vi "SatelliteTracking.vi"() -> ()   [LabVIEW 2014]
uses:
  <vilib>/Analysis/NI_AALBase.lvlib
  <vilib>/measure/NI_MAPro.lvlib
  <vilib>/measure/maspectr.llb/FFT Power Spectrum and PSD for 1 Chan.vi
  <vilib>/Analysis/4window.llb/windowTd.ctl
  <vilib>/Analysis/NI_AALPro.lvlib
panel:
  in  "dB On (F)":bool
  in  "window parameter":dbl=nan
  in  "window":T1=1 items=["Rectangle"=0, "Hanning"=1, "Hamming"=2, "Blackman-Harris"=3, "Exact Blackman"=4, "Blackman"=5, "Flat Top"=6, "4 Term B-Harris "=7, "7 Term B-Harris"=8, "Low Sidelobe"=9, "Blackman Nuttall"=11, "Triangle"=30, "Bartlett-Hanning"=31, "Bohman"=32, "Parzen"=33, "Welch"=34, "Kaiser"=60, "Dolph-Chebyshev"=61, "Gaussian"=62]
  in  "averaging parameters":T2={"averaging mode"=enum."No averaging", "weighting mode"=enum."Exponential", "number of averages"=10} {"number of averages" min=1}
  out "Power Spectrum":cluster{"f0":dbl, "df":dbl, "magnitude":dbl[]}(graph)
  in  "frequency":dbl=0.0078125 format="%0.4e"
  in  "amplitude":dbl=1.0 format="%0.2f"
  in  "samples":i32=128
  in  "Longitude":dbl=-1.307 format="%#.6g"
  in  "Latitude":dbl=51.4062 format="%#.6g"
  out "URL":string="http://maps.google.com/staticmap?center=51.406200,-1.307000&zoom=18&size=570x350&maptype=hybrid&markers=51.406200,-1.307000,midpurplea&key=&path=rgb:0xFF1000,weight:5|51.406200,-1.307000|51.406200,-1.307000"
  in  "?":refnum<k7>(container)
  # "Start Position"
  # "Balloon Position"
  # "This is an 86 character alphanumeric key supplied by Google"
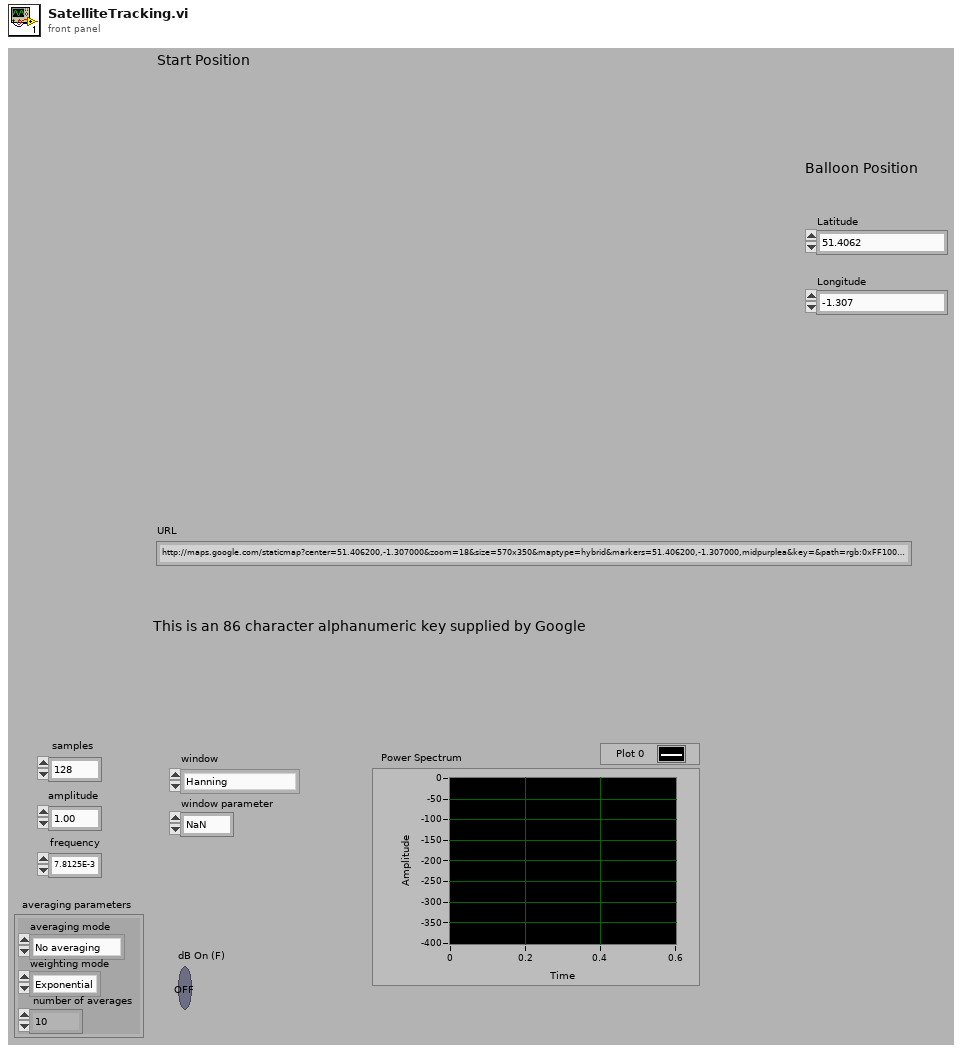
[diagram p1: front panel]
types:
  T1 = typedef "NI_AALPro.lvlib/windowTd.ctl" = u32
  T2 = cluster{"averaging mode":enum16{"No averaging", "Vector averaging", "RMS averaging", "Peak hold"}, "weighting mode":enum16{"Linear", "Exponential"}, "number of averages":u32}
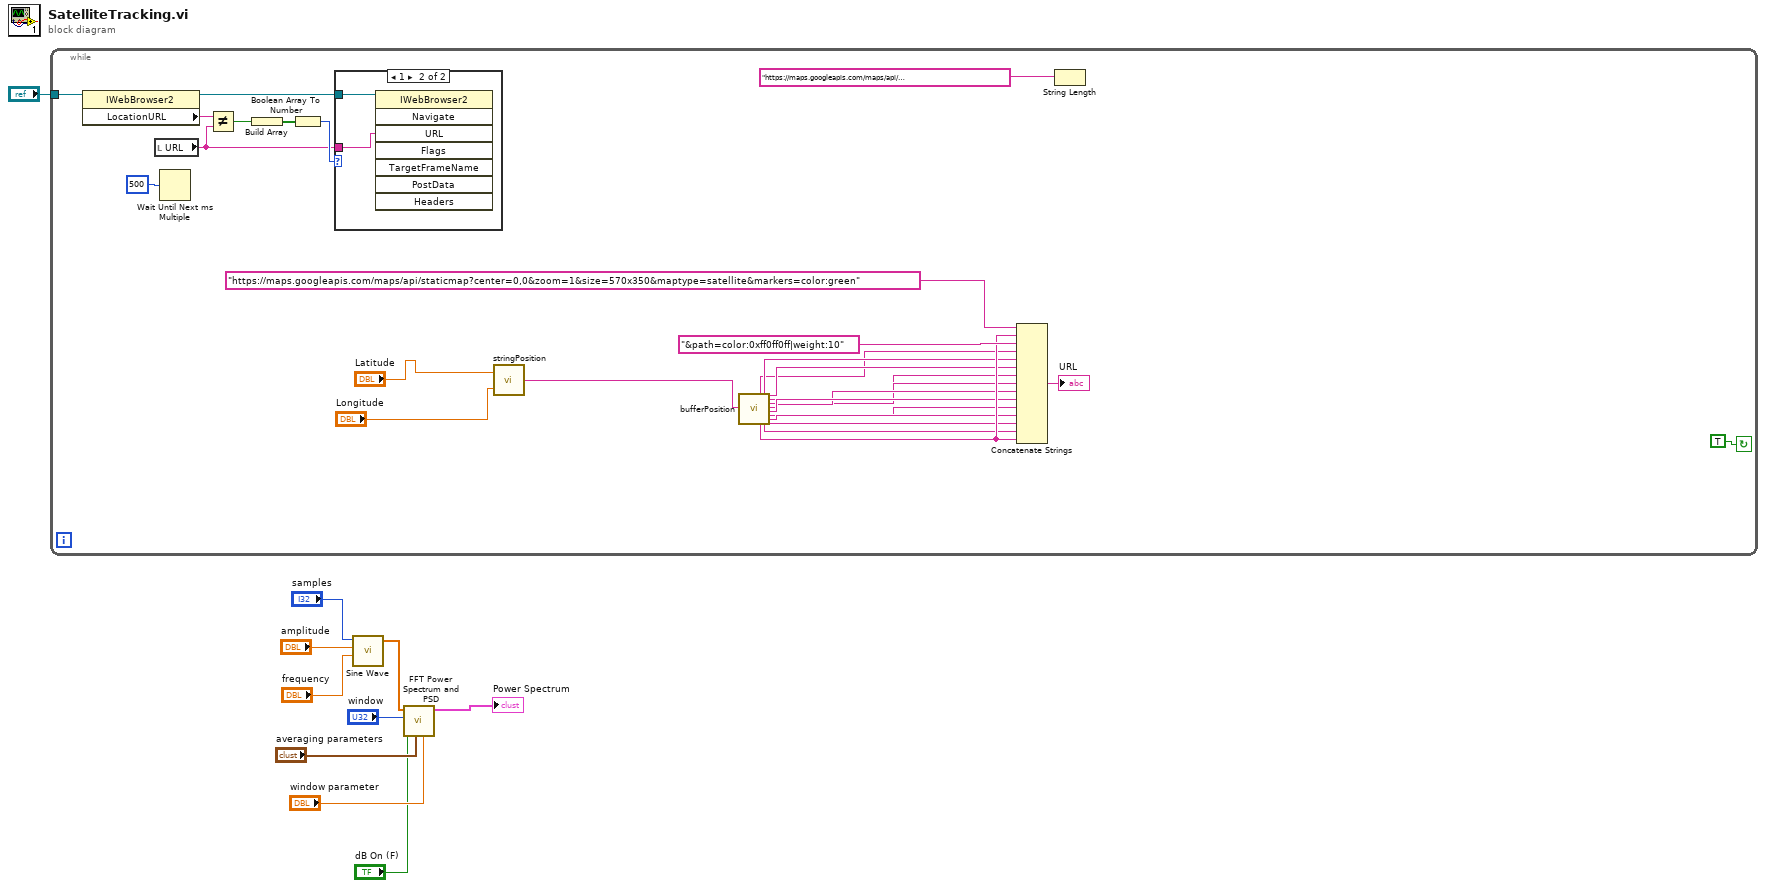
[diagram p0: block diagram]
diagram:
  n1 = while {
    tunnel: "?" -> [w36]
    stop <- TRUE continue-if-true
    n2 = property class="IWebBrowser2"(reference=w36) -> (reference out=w35:refnum<k7>, "LocationURL"=w33:string)  [unwired: 1 in, 1 out]
    n3 = local read "URL"() -> (w28:string)
    n4 = Wait Until Next ms Multiple(millisecond multiple=u32 500) -> ()  [unwired: 1 out]
    n5 = Not Equal?(x=w33, y=w28) -> (x != y?=w34:bool)
    n6 = Build Array(w34) -> (w32:bool[])
    n7 = Boolean Array To Number(Boolean array=w32) -> (number=w31:u32)
    n8 = case shown="1" w31 {
      tunnel: w28 -> [_ w40]
      tunnel: w35 -> [_ w39]
      frame 0, Default {
      }
      frame 1 {
        n9 = invoke class="IWebBrowser2" method="Navigate"(reference=w39, "URL"=w40) -> ()  [unwired: 6 in, 8 out]
      }
    }
    n10 = call "stringPosition.vi"("Longitude"="Longitude", "Latitude"="Latitude") -> ("StringPosition"=w23:string)
    n11 = call "bufferPosition.vi"("Input String"=w23) -> ("Output 12"=w11:string, "Output1"=w22:string, "Output 11"=w12:string, "Output 2"=w21:string, "Output 10"=w13:string, "Output 9"=w14:string, "Output 8"=w15:string, "Output 7"=w16:string, "Output 6"=w17:string, "Output 5"=w18:string, "Output 4"=w19:string, "Output 3"=w20:string)  [unwired: 15 in]
    n12 = Concatenate Strings("https://maps.googleapis.com/maps/api/staticmap?center=0,0&zoom=1&size=570x350&maptype=satellite&markers=color:green" ("URL"), w22, "&path=color:0xff0ff0ff|weight:10", w11, w12, w13, w14, w15, w16, w17, w18, w19, w20, w21, w22) -> (→"URL":string)
    n13 = String Length(string="https://maps.googleapis.com/maps/api/staticmap?center=0,0&zoom=1&size=570x350&maptype=satellite&markers=color:green|49.926586,15.405640&path=color:0xff0ff0ff|weight:10|50.737102,15.400318|40.749825,-73.987963|60.752946,-63.987384|40.755823,-73.986397") -> ()  [unwired: 1 out]
  }
  n14 = call <vilib>:"Sine Wave.vi"("samples"="samples", "amplitude"="amplitude", "frequency"="frequency") -> ("sine wave"=w6:dbl[])  [unwired: 2 in, 2 out]
  n15 = call-poly <vilib>:"FFT Power Spectrum and PSD.vi"("window parameter"="window parameter", "averaging parameters"="averaging parameters", "dB On (F)"="dB On (F)", "window"="window", "time signal"=w6) -> ("Power Spectrum / PSD"=→"Power Spectrum":cluster{"f0":dbl, "df":dbl, "magnitude":dbl[]})  [unwired: 3 in, 3 out]
